vi "Hardware-SkipFireSetupCalPoints.vi"(11 "Skipfire Setup":T1[](array[typedef])) -> (3 "Skipfire Setup":T1[](array[typedef]))   [LabVIEW 2016, in "DSI-RT.lvlib"]
uses:
  DSI-RT.lvlib
  <vilib>/Powertrain Controls/Device Drivers/DCM/Skip Fire/RT/Skip Fire Setup.ctl
  <vilib>/addons/Software Calibration Management/xSCM/CalPoint.xnode
  <vilib>/addons/Software Calibration Management/xSCM/ni_scm.dll
  <vilib>/Powertrain Controls/Device Drivers/DCM/Skip Fire/RT/DCM - RT - Skip Fire.lvlib
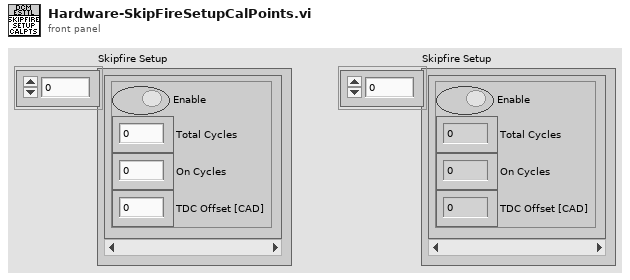
[diagram p1: front panel]
types:
  T1 = typedef "DCM - RT - Skip Fire.lvlib/Skip Fire Setup.ctl" = cluster{"Enable":bool, "Total Cycles":u8, "On Cycles":u8, "TDC Offset [CAD]":sgl}
  T2 = cluster{"Enable":bool, "Total Cycles":u8, "On Cycles":u8, "TDC Offset [CAD]":sgl}[]
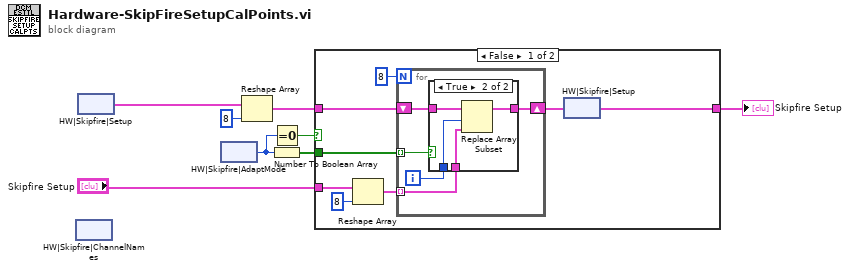
[diagram p0: block diagram]
diagram:
  n1 = xnode "HW|Skipfire|ChannelNames"() -> ()  [unwired: 1 out]
  n2 = xnode "HW|Skipfire|Setup"() -> ("Value"=w1:T2)
  n3 = xnode "HW|Skipfire|AdaptMode"() -> ("Value"=w5:u32)
  n4 = Reshape Array(w1, 8 ("dimension size")) -> (w8:T2)
  n5 = Equal To 0?(x=w5) -> (x = 0?=w4:bool)
  n6 = Number To Boolean Array(number=w5) -> (Boolean array=w6:bool[])
  n7 = case shown="False" w4 {
    tunnel: w8 -> [w15 w31]
    tunnel: [w9 w31] -> w2
    tunnel: w6 -> [w13 _]
    tunnel: "Skipfire Setup" -> [w10 _]
    frame False {
      n8 = Reshape Array(w10, 8 ("dimension size")) -> (w11:T1[])
      n9 = for {
        N: 8 -> [_]
        tunnel: w13 -> [w21] mode=indexing
        shift-right: [w24] -> w9
        shift-left: w15 -> [w25]
        tunnel: w11 -> [w22] mode=indexing
        i -> [w23]
        n10 = case shown="True" w21 {
          tunnel: w25 -> [w26 w30]
          tunnel: [w26 w29] -> w24
          tunnel: w23 -> [_ w28]
          tunnel: w22 -> [_ w27]
          frame False {
          }
          frame True {
            n11 = Replace Array Subset(array=w30, new element=w27, index=w28) -> (w29:T2)
          }
        }
      }
      n12 = xnode "HW|Skipfire|Setup"("Value"=w9) -> ()
    }
    frame True {
    }
  }
  "Skipfire Setup" <- w2
